vi "Get Fields.vi"(11 "Device Info in":refnum<class "Device Info.lvclass">) -> (2 "Fields":variant[](array[variant]), 3 "Device Info out":refnum<class "Device Info.lvclass">)   [LabVIEW 2019, in "Electronic Datasheet.lvlib" / "Device Info.lvclass"]
uses:
  Device Info.lvclass
  Device Info.lvclass/Device Info.ctl
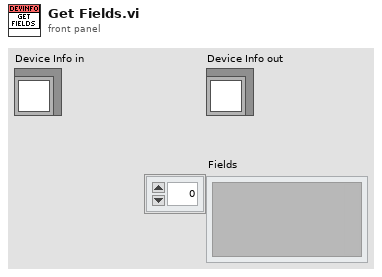
[diagram p1: front panel]
types:
  T1 = cluster{"VendorName":string, "VendorNumber":u32, "ProductName":string, "ProductNumber":u32, "RevisionNumber":u32, "OrderCode":string, "BaudRate_10":bool, "BaudRate_20":bool, "BaudRate_50":bool, "BaudRate_125":bool, "BaudRate_250":bool, "BaudRate_500":bool, "BaudRate_800":bool, "BaudRate_1000":bool, "BaudRate_auto":bool, "SimpleBootUpMaster":bool, "SimpleBootUpSlave":bool, "Granularity":u8, "DynamicChannelsSupported":bool, "CompactPDO":u8, "GroupMessaging":bool, "NrOfRXPDO":u16, "NrOfTXPDO":u16, "LSS_Supported":bool, "LSS_Master":bool, "NG_Slave":bool, "NG_Master":bool, "NrOfNG_MonitoredNodes":u16}
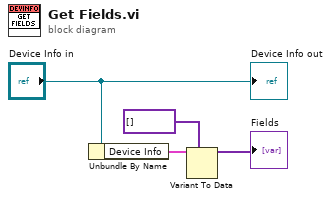
[diagram p0: block diagram]
diagram:
  n1 = Unbundle By Name("Device Info in") -> ("Device Info"=w3:T1)
  n2 = Variant To Data(type=variant[] [], Variant=w3) -> (data=→"Fields":variant[])  [unwired: 1 in, 1 out]
  "Device Info out" <- "Device Info in"
